vi "blank_background.vi"(5 "plots":u32(colorbox)=13816530, 7 "backg":u32(colorbox)=13816530, 8 "error in (no error)":errorcluster, 9 "plots":refnum<vi>, 10 "experiments 2":refnum<vi>, 11 "VI in":refnum<vi>) -> (0 "error in (no error) 2":errorcluster)   [LabVIEW 2018]
uses:
  <vilib>/picture/picture.llb/imagedata.ctl
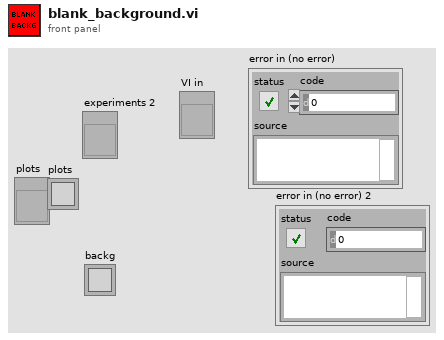
[diagram p1: front panel]
types:
  T1 = typedef "imagedata.ctl" = cluster{"image type":i32, "image depth":i32, "image":u8[], "mask":u8[], "colors":u32[], "Rectangle":cluster{"left":i16, "top":i16, "right":i16, "bottom":i16}}
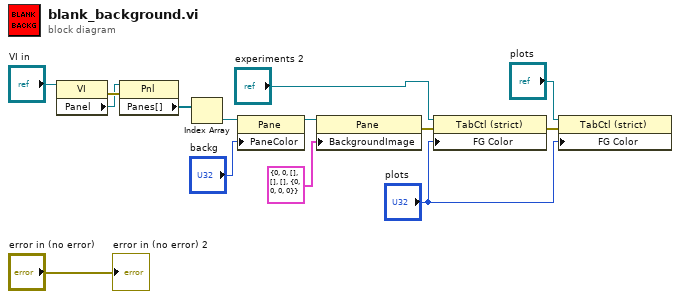
[diagram p0: block diagram]
diagram:
  n1 = property class="VI"(reference="VI in") -> (error out=w10:errorcluster, "Panel"=w9:refnum<vi>)  [unwired: 1 in, 1 out]
  n2 = property class="Pnl"(reference=w9, error in=w10) -> ("Panes[]"=w11:refnum<vi>[])  [unwired: 2 out]
  n3 = Index Array(array=w11) -> (element=w12:refnum<vi>)  [unwired: 1 in]
  n4 = property class="Pane"(reference=w12, "PaneColor"="backg") -> (reference out=w13:refnum<vi>)  [unwired: 1 in, 1 out]
  n5 = property on="Property Node" class="Pane"(reference=w13, "BackgroundImage"=T1 {"image type"=0, "image depth"=0, "image"=[], "mask"=[], "colors"=[], "Rectangle"={"left"=0, "top"=0, "right"=0, "bottom"=0}} ("Background Image")) -> (error out=w5:errorcluster)  [unwired: 1 in, 1 out]
  n6 = property class="TabCtl (strict)"(reference="experiments 2", error in=w5, "FG Color"="plots") -> (error out=w6:errorcluster)  [unwired: 1 out]
  n7 = property class="TabCtl (strict)"(reference="plots", error in=w6, "FG Color"="plots") -> ()  [unwired: 2 out]
  "error in (no error) 2" <- "error in (no error)"
